vi "Handle Last Ack Core.vi"(4 "error in (no error)":errorcluster, 6 "Last Ack":refnum<class "Last Ack.lvclass">, 7 "Controller in":refnum<class "Controller.lvclass">) -> (0 "error out":errorcluster, 3 "Controller out":refnum<class "Controller.lvclass">)   [LabVIEW 2026, in "Controller Actor.lvlib" / "Controller.lvclass"]
doc: "(<B>Filename</B>: Actor Framework.lvlib:Actor.lvclass:Handle Last Ack Core.vi)\n\nDefines how the caller actor responds to the Last Ack message from a nested actor. The Last Ack message is the final message a nested actor sends to its caller before it shuts down. The message contains information about the final state of the nested actor.\n\nBy default, this method does nothing except return any error the nested actor sent. A descendant class may override this method to define behavior."
uses:
  Controller.lvclass
  <vilib>/ActorFramework/LastAck/Last Ack.lvclass
  C:/Program Files/National Instruments/LabVIEW 2026/vi.lib/ActorFramework/Actor/Actor.lvclass
  <vilib>/ActorFramework/LastAck/Last Ack.lvclass/Last Ack.ctl
  Hardware/HW Config/HW Configuration.lvclass
  C:/Users/E2013170/Documents/GitHub/Measurement-Utility-Reference/source/configuration/Configuration.lvclass
  <vilib>/ActorFramework/Actor/Actor.lvclass/Actor.ctl
  <vilib>/ActorFramework/Message Enqueuer/Message Enqueuer.lvclass/Message Enqueuer.ctl
  Hardware/HW Config/HW Configuration.lvclass/HW Configuration.ctl
  Controller Messages/Apply Hardware Configurations Msg/Apply Hardware Configurations Msg.lvclass/Apply Hardware Configurations Msg.ctl
  Measurement Actor/Configuration/Step Configuration.lvclass
  Measurement Actor/Configuration/Step Configuration.lvclass/Step Configuration.ctl
  Controller Messages/Apply Step Configuration Msg/Apply Step Configuration Msg.lvclass/Apply Step Configuration Msg.ctl
  configuration/Configuration.lvclass
  Controller.lvclass/Controller.ctl
  Measurement Actor/Measurement.lvclass
  Measurement Actor/Measurement.lvclass/Measurement.ctl
  <vilib>/ActorFramework/Message Enqueuer/Init from Existing Queue.vi
  <vilib>/ActorFramework/Message Enqueuer/Enqueue.vi
  Controller Messages/Apply Hardware Configurations Msg/Apply Hardware Configurations Msg.lvclass
  C:/Program Files/National Instruments/LabVIEW 2026/vi.lib/ActorFramework/Message/Message.lvclass
  Controller Messages/Apply Step Configuration Msg/Apply Step Configuration Msg.lvclass
  User Interface/Messages/Enable UI Msg/Enable UI Msg.lvclass
  <vilib>/ActorFramework/Message Priority Queue/Priority Enqueue.vi
  <vilib>/ActorFramework/Actor/Actor.lvclass
  <vilib>/ActorFramework/Message Enqueuer/Message Enqueuer.lvclass
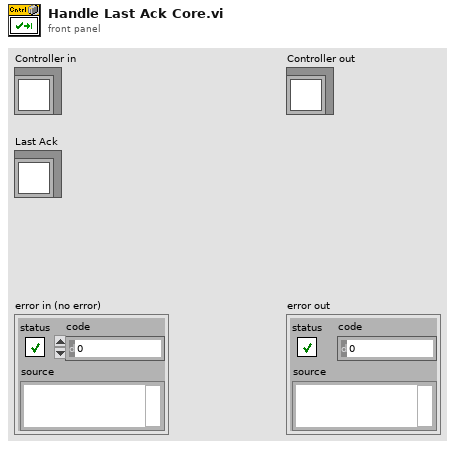
[diagram p1: front panel]
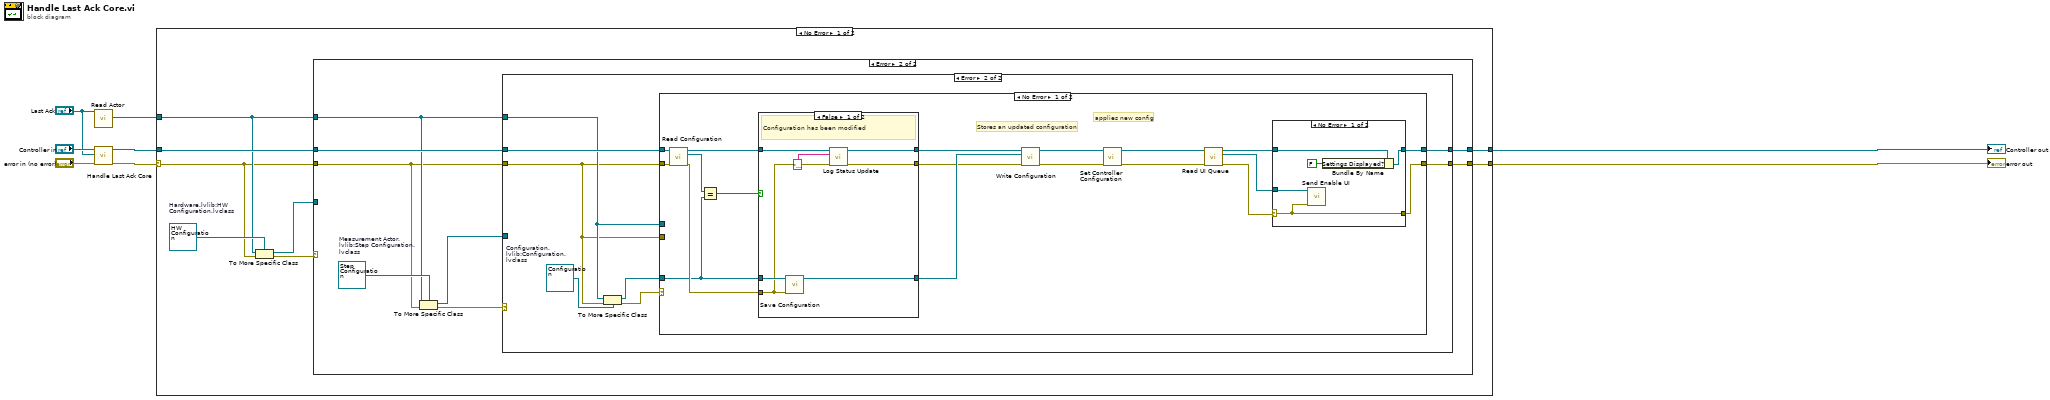
[diagram p0: block diagram]
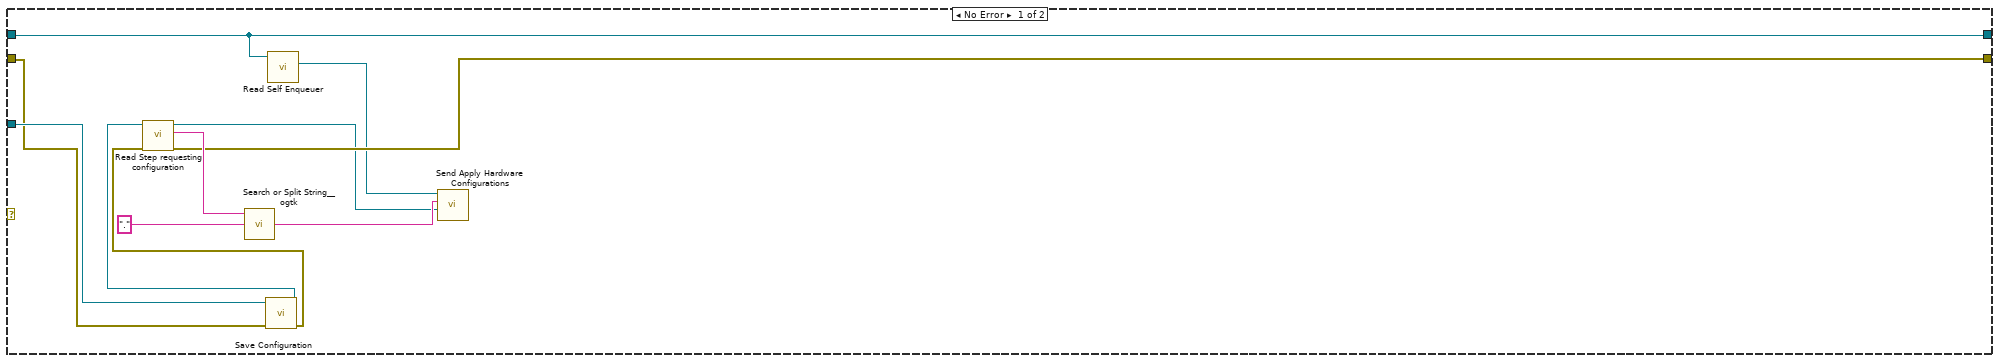
[diagram p2: hidden frame]
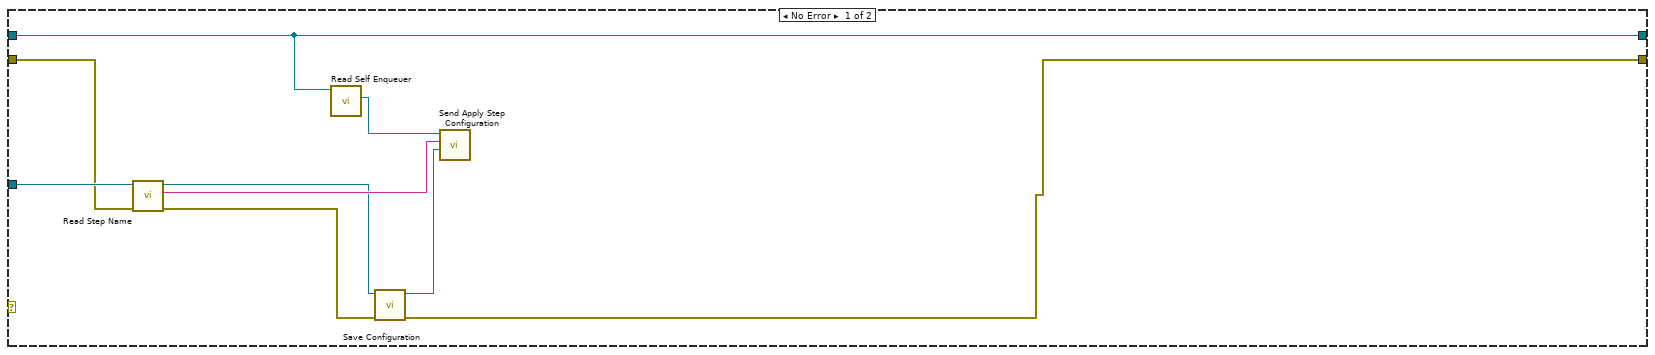
[diagram p3: hidden frame]
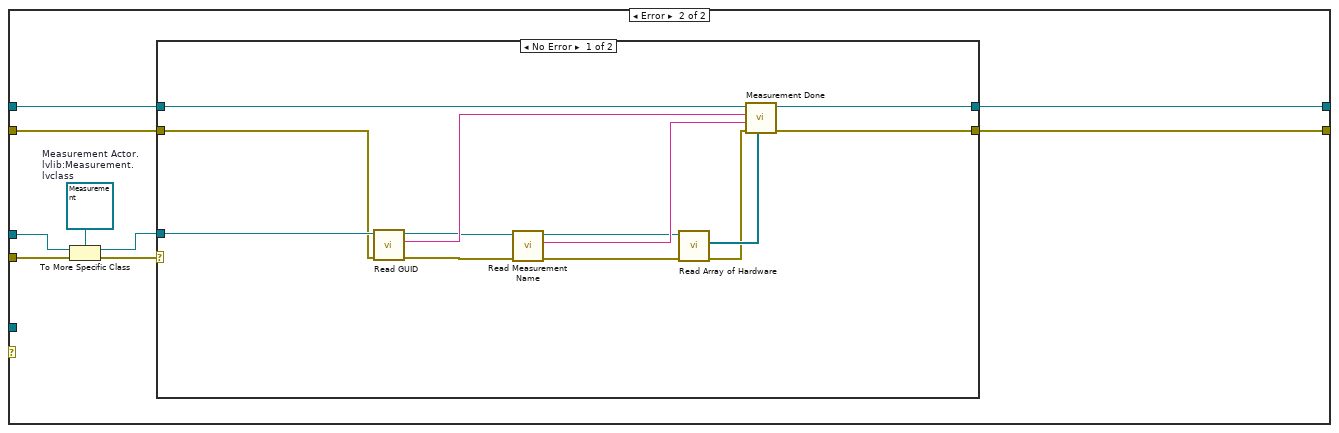
[diagram p6: hidden frame]
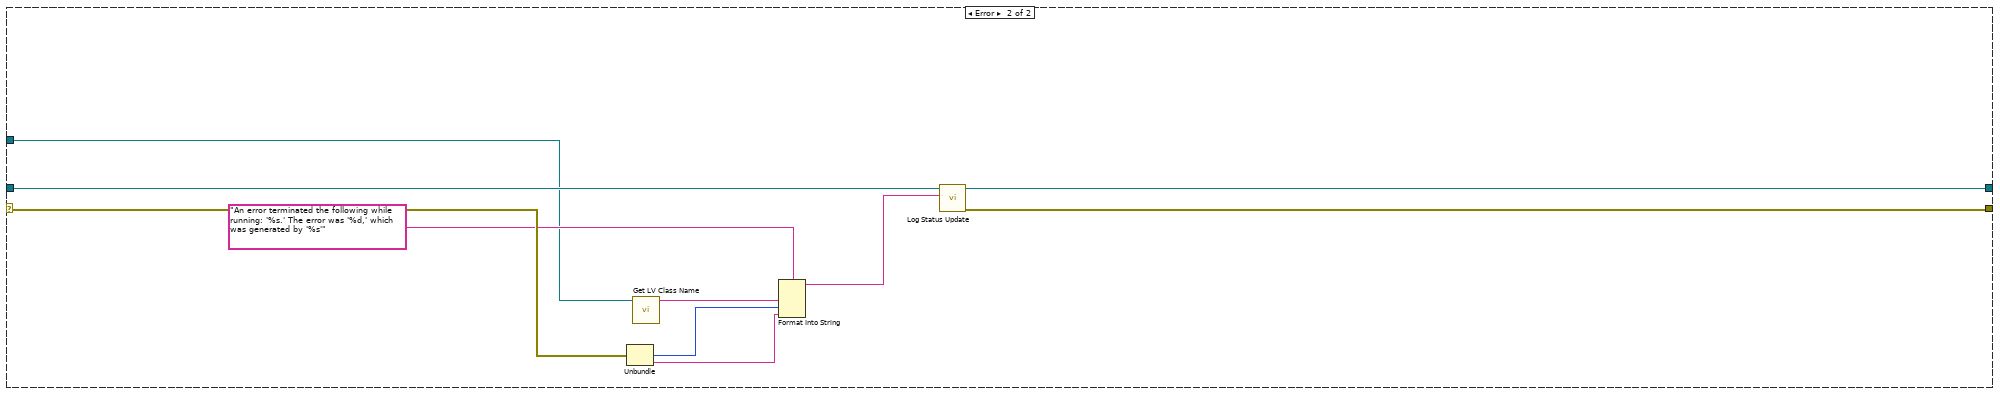
[diagram p8: hidden frame]
diagram:
  n1 = call <vilib>:"Read Actor.vi"("Last Ack"="Last Ack") -> ("Actor"=w2:refnum<class "Actor.lvclass">)  [unwired: 10 in]
  n2 = call-parent "Handle Last Ack Core.vi"("error in (no error)"="error in (no error)", "Last Ack"="Last Ack", "Actor in"="Controller in") -> ("error out"=w1:errorcluster, "Actor out"=w4:refnum<class "Controller.lvclass">)  [unwired: 3 in]
  n3 = case shown="No Error" w1 {
    selector: w1 -> [w9 w118]
    tunnel: [w16 w121] -> w7
    tunnel: [w15 w120] -> w5
    tunnel: w4 -> [w14 w122]
    tunnel: w2 -> [w12 w114]
    frame No Error {
      w13 = refnum<class "HW Configuration.lvclass"> refnum  # Hardware.lvlib:HW Configuration.lvclass
      n4 = To More Specific Class(target class=w13, reference=w12, error in=w9) -> (specific class reference=w11:refnum<class "HW Configuration.lvclass">, error out=w10:errorcluster)
      n5 = case shown="Error" w10 {
        tunnel: [w25 w35] -> w16
        tunnel: [w24 w34] -> w15
        tunnel: w14 -> [w25 w33]
        tunnel: w12 -> [_ w31]
        tunnel: w9 -> [w19 w29]
        tunnel: w11 -> [w20 _]
        frame No Error {
          n6 = call "Save Configuration.vi"("error in (no error)"=w19, "Configuration in"=w20) -> ("error out"=w18:errorcluster, "Configuration out"=w17:refnum<class "HW Configuration.lvclass">)  [unwired: 7 in, 1 out]
          n7 = call "Read Step requesting configuration.vi"("error in (no error)"=w18, "HW Configuration in"=w17) -> ("error out"=w24:errorcluster, "Step requesting configuration"=w26:string, "HW Configuration out"=w21:refnum<class "HW Configuration.lvclass">)  [unwired: 7 in]
          n8 = call <userlib>:"Search or Split String__ogtk.vi"("search string/char (-)"="." ("regular expression"), "string"=w26) -> ("substring after match"=w22:string)  [unwired: 1 in, 2 out]
          n9 = call <vilib>:"Read Self Enqueuer.vi"("Actor"=w25) -> ("Self Enqueuer"=w23:refnum<class "Message Enqueuer.lvclass">)  [unwired: 10 in]
          n10 = call "Send Apply Hardware Configurations.vi"("HW Config Object"=w21, "Device Name"=w22, "Message Enqueuer"=w23) -> ()  [unwired: 7 in, 2 out]
        }
        frame Error {
          w32 = refnum<class "Step Configuration.lvclass"> refnum  # Measurement Actor.lvlib:Step Configuration.lvclass
          n11 = To More Specific Class(target class=w32, reference=w31, error in=w29) -> (specific class reference=w28:refnum<class "Step Configuration.lvclass">, error out=w30:errorcluster)
          n12 = case shown="Error" w30 {
            tunnel: [w40 w52] -> w35
            tunnel: [w37 w51] -> w34
            tunnel: w33 -> [w40 w50]
            tunnel: w31 -> [_ w46]
            tunnel: w29 -> [w43 w45]
            tunnel: w28 -> [w44 _]
            frame No Error {
              n13 = call "Read Step Name.vi"("error in (no error)"=w43, "Step Configuration in"=w44) -> ("error out"=w38:errorcluster, "Step Name"=w42:string, "Step Configuration out"=w39:refnum<class "Step Configuration.lvclass">)  [unwired: 7 in]
              n14 = call <vilib>:"Read Self Enqueuer.vi"("Actor"=w40) -> ("Self Enqueuer"=w41:refnum<class "Message Enqueuer.lvclass">)  [unwired: 10 in]
              n15 = call "Save Configuration.vi"("error in (no error)"=w38, "Configuration in"=w39) -> ("error out"=w37:errorcluster, "Configuration out"=w36:refnum<class "Step Configuration.lvclass">)  [unwired: 7 in, 1 out]
              n16 = call "Send Apply Step Configuration.vi"("Measurement Actor.lvlib:Step Configuration.lvclass"=w36, "Measurement Name"=w42, "Message Enqueuer"=w41) -> ()  [unwired: 7 in, 2 out]
            }
            frame Error {
              w47 = refnum<class "Configuration.lvclass"> refnum  # Configuration.lvlib:Configuration.lvclass
              n17 = To More Specific Class(target class=w47, reference=w46, error in=w45) -> (specific class reference=w49:refnum<class "Configuration.lvclass">, error out=w48:errorcluster)
              n18 = case shown="No Error" w48 {
                tunnel: [w66 w90] -> w52
                tunnel: [w63 w89] -> w51
                tunnel: w50 -> [w61 w92]
                tunnel: w49 -> [w58 _]
                tunnel: w45 -> [w56 w91]
                tunnel: w46 -> [_ w97]
                tunnel: w45 -> [_ w96]
                frame No Error {
                  # "applies new config"
                  # "Stores an updated configuration"
                  n19 = call "Read Configuration.vi"("error in (no error)"=w56, "Controller in"=w61) -> ("error out"=w60:errorcluster, "Configuration.lvlib:Configuration.lvclass"=w59:refnum<class "Configuration.lvclass">, "Controller out"=w55:refnum<class "Controller.lvclass">)  [unwired: 7 in]
                  n20 = Equal?(x=w59, y=w58) -> (x = y?=w57:bool)
                  n21 = case shown="False" w57 {
                    tunnel: w58 -> [w78 w81]
                    tunnel: [w77 w81] -> w62
                    tunnel: w60 -> [w73 w79]
                    tunnel: w55 -> [w76 w80]
                    tunnel: [w75 w80] -> w54
                    tunnel: [w72 w79] -> w53
                    frame False {
                      # "Configuration has been modified"
                      n22 = call "Save Configuration.vi"("error in (no error)"=w73, "Configuration in"=w78) -> ("Configuration out"=w77:refnum<class "Configuration.lvclass">)  [unwired: 7 in, 2 out]
                      n23 = call-dynamic "Log Status Update.vi"("error in (no error)"=w73, "String"="Settings updated and saved to disk without error", "Controller in"=w76) -> ("error out"=w72:errorcluster, "Controller out"=w75:refnum<class "Controller.lvclass">)  [unwired: 7 in]
                    }
                    frame True {
                    }
                  }
                  n24 = call "Write Configuration.vi"("error in (no error)"=w53, "Configuration.lvlib:Configuration.lvclass"=w62, "Controller in"=w54) -> ("error out"=w71:errorcluster, "Controller out"=w70:refnum<class "Controller.lvclass">)  [unwired: 7 in]
                  n25 = call-dynamic "Set Controller Configuration.vi"("error in (no error)"=w71, "Controller in"=w70) -> ("error out"=w65:errorcluster, "Controller out"=w69:refnum<class "Controller.lvclass">)  [unwired: 8 in]
                  n26 = call "Read UI Queue.vi"("error in (no error)"=w65, "UI Controller in"=w69) -> ("error out"=w64:errorcluster, "UI Queue"=w68:refnum<class "Message Enqueuer.lvclass">, "UI Controller out"=w67:refnum<class "Controller.lvclass">)  [unwired: 7 in]
                  n27 = case shown="No Error" w64 {
                    selector: w64 -> [w82 w87]
                    tunnel: w68 -> [w86 _]
                    tunnel: w67 -> [w85 w88]
                    tunnel: [w83 w88] -> w66
                    tunnel: [w82 w87] -> w63
                    frame No Error {
                      n28 = call "Send Enable UI.vi"("error in (no error)"=w82, "Message Enqueuer"=w86) -> ()  [unwired: 8 in, 2 out]
                      n29 = Bundle By Name(cluster=w85, "Settings Displayed?"=FALSE) -> (w83:refnum<class "Controller.lvclass">)
                    }
                    frame Error {
                    }
                  }
                }
                frame Error {
                  w95 = refnum<class "Measurement.lvclass"> refnum  # Measurement Actor.lvlib:Measurement.lvclass
                  n30 = To More Specific Class(target class=w95, reference=w97, error in=w96) -> (specific class reference=w93:refnum<class "Measurement.lvclass">, error out=w94:errorcluster)
                  n31 = case shown="No Error" w94 {
                    tunnel: w93 -> [w104 _]
                    tunnel: w92 -> [w110 w112]
                    tunnel: w91 -> [w100 w111]
                    tunnel: [w109 w112] -> w90
                    tunnel: [w108 w111] -> w89
                    frame No Error {
                      n32 = call "Read GUID.vi"("error in (no error)"=w100, "Measurement in"=w104) -> ("error out"=w99:errorcluster, "GUID"=w106:string, "Measurement out"=w103:refnum<class "Measurement.lvclass">)  [unwired: 7 in]
                      n33 = call "Read Measurement Name.vi"("error in (no error)"=w99, "Measurement in"=w103) -> ("error out"=w98:errorcluster, "Measurement Name"=w105:string, "Measurement out"=w102:refnum<class "Measurement.lvclass">)  [unwired: 7 in]
                      n34 = call "Read Array of Hardware.vi"("error in (no error)"=w98, "Measurement in"=w102) -> ("error out"=w101:errorcluster, "Array of Hardware"=w107:refnum<class "Hardware.lvclass">[])  [unwired: 7 in, 1 out]
                      n35 = call-dynamic "Measurement Done.vi"("Array of Hardware"=w107, "error in (no error)"=w101, "Measurement Name"=w105, "GUID"=w106, "Controller in"=w110) -> ("error out"=w108:errorcluster, "Controller out"=w109:refnum<class "Controller.lvclass">)  [unwired: 5 in]
                    }
                    frame Error {
                    }
                  }
                }
              }
            }
          }
        }
      }
    }
    frame Error {
      # "No actor that the controller launches should be able to shut\ndown the controller, which is why all errors are cleared here"
      n36 = Unbundle(w118) -> ("code"=w116:i32, "source"=w115:string)  [unwired: 1 out]
      n37 = call <vilib>:"Get LV Class Name.vi"("object"=w114) -> ("class name"=w113:string)  [unwired: 9 in, 1 out]
      n38 = Format Into String(format string="An error terminated the following while running: '%s.' The error was '%d,' which was generated by '%s'", w113, w116, w115) -> (resulting string=w119:string)  [unwired: 2 in, 1 out]
      n39 = call-dynamic "Log Status Update.vi"("String"=w119, "Controller in"=w122) -> ("error out"=w120:errorcluster, "Controller out"=w121:refnum<class "Controller.lvclass">)  [unwired: 8 in]
    }
  }
  "Controller out" <- w7
  "error out" <- w5
